vi "PhotonCamera_GetLatestResult_OLD.vi"(6 "EstimatedDataAndSampleLatency (Sec)":dbl=0.05 format="%#_13g", 8 "Pass_Through_Time":dbl=-1.0 format="%33.4f", 9 "BaseNTName":string="/photonvision", 11 "CameraName":string) -> (0 "error out":errorcluster, 1 "New Data":bool, 2 "HasTargets":bool, 3 "PipelineResult":T1={"Targets"=[], "PhotonMultiTargetPNPResult"={"PhotonPNPResult"={"IsPresent"=FALSE, "bestReprojErr"=0.0, "altReprojErr"=0.0, "ambiguity"=0.0, "Best"={"TRANSLATION3D"={"X"=0.0, "Y"=0.0, "Z"=0.0}, "ROTATION3D"={"Q_quaternion"={"R"=1.0, "V"=[0.0, 0.0, 0.0]}}, "XF"=FALSE}, "Alt"={"TRANSLATION3D"={"X"=0.0, "Y"=0.0, "Z"=0.0}, "ROTATION3D"={"Q_quaternion"={"R"=1.0, "V"=[0.0, 0.0, 0.0]}}, "XF"=FALSE}}, "FiducialIDsUsed"=[]}, "PhotonPipelineMetadata"={"CaptureTimestampMicros"=0, "PublishTimestampMicros"=0, "SequenceID"=0, "TimeSinceLastPong"=0}} {"PhotonMultiTargetPNPResult"."PhotonPNPResult"."Alt"."TRANSLATION3D"."Z" format="%14.3f"; "PhotonMultiTargetPNPResult"."PhotonPNPResult"."Alt"."TRANSLATION3D"."Y" format="%14.3f"; "PhotonMultiTargetPNPResult"."PhotonPNPResult"."Alt"."TRANSLATION3D"."X" format="%14.3f"; "PhotonMultiTargetPNPResult"."PhotonPNPResult"."Best"."TRANSLATION3D"."Z" format="%14.3f"; "PhotonMultiTargetPNPResult"."PhotonPNPResult"."Best"."TRANSLATION3D"."Y" format="%14.3f"; "PhotonMultiTargetPNPResult"."PhotonPNPResult"."Best"."TRANSLATION3D"."X" format="%14.3f"; "Targets"."AltCameraToTarget"."TRANSLATION3D"."Z" format="%14.3f"; "Targets"."AltCameraToTarget"."TRANSLATION3D"."Y" format="%14.3f"; "Targets"."AltCameraToTarget"."TRANSLATION3D"."X" format="%14.3f"; "Targets"."BestCameraToTarget"."TRANSLATION3D"."Z" format="%14.3f"; "Targets"."BestCameraToTarget"."TRANSLATION3D"."Y" format="%14.3f"; "Targets"."BestCameraToTarget"."TRANSLATION3D"."X" format="%14.3f"})   [LabVIEW 2019, in "PhotonVisionLib.lvlib"]
doc: "Returns the latest pipeline result.\n\nInputs:\n - cameraName -- The nickname of the camera (found in the PhotonVision UI).\n - BaseNTName - string - Base Nework Table name. (Optional. Default: /photonvision )\n - PassThroughTime -- (Optional. Default: Use FPGA time.) Time. Once time is available from network tables, this won't be needed. (Seconds)\n - EstimatedDataAndSampleLatency -- Estimated Network Table packet latency. This is based on the frames per second and other communications latencies. (Optional. Default: 0.050) Once time is available from network tables, this won't be needed. \n\nOutputs:\n - PipelineResult -- The latest pipeline result data cluster\n - HasTargets -- Boolean indicating if any targets were found\n - Error Out -- Contains error information if a Network table ot other error occured."
uses:
  PhotonVisionLib.lvlib
  <vilib>/Rock Robotics/Network Tables/NT Read Raw.vi
  <vilib>/Rock Robotics/WPI/ThirdParty/JAS_Junk/TrajLib/Trajectory_Library.lvlib
  TypeDef/TargetCornerType.ctl
  TypeDef/PhotonTrackedTargetType.ctl
  TypeDef/PhotonPipelineResultType.ctl
  <vilib>/Rock Robotics/WPI/ThirdParty/JAS_Junk/TrajLib/TypeDef/TRANSLATION3D.ctl
  <vilib>/Rock Robotics/WPI/ThirdParty/JAS_Junk/TrajLib/TypeDef/QUATERNION.ctl
  <vilib>/Rock Robotics/WPI/ThirdParty/JAS_Junk/TrajLib/TypeDef/ROTATION3D.ctl
  <vilib>/Rock Robotics/WPI/ThirdParty/JAS_Junk/TrajLib/TypeDef/TRANSFORM3D.ctl
  TypeDef/PhotonPNPResultType.ctl
  TypeDef/PhotonMultiTargetPNPResultType.ctl
  TypeDef/PhotonPipelineMetadataType.ctl
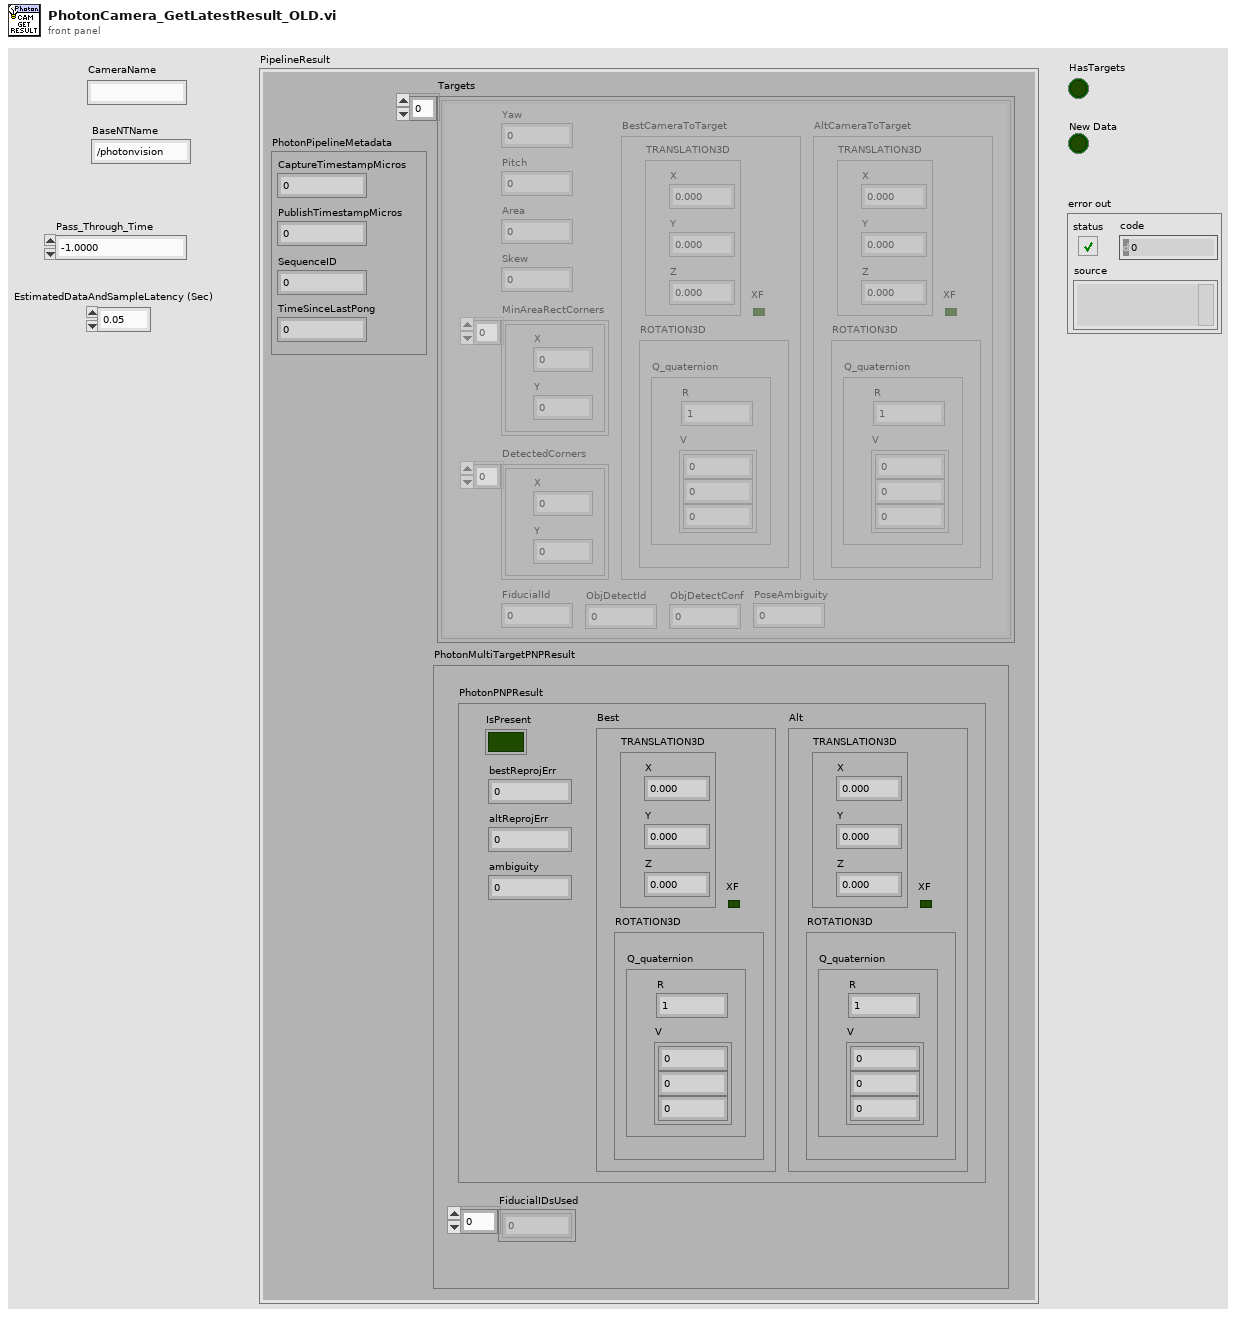
[diagram p1: front panel]
types:
  T1 = typedef "PhotonVisionLib.lvlib/PhotonPipelineResultType.ctl" = cluster{"Targets":T2[], "PhotonMultiTargetPNPResult":T8, "PhotonPipelineMetadata":T10}
  T2 = typedef "PhotonVisionLib.lvlib/PhotonTrackedTargetType.ctl" = cluster{"Yaw":dbl, "Pitch":dbl, "Area":dbl, "Skew":dbl, "MinAreaRectCorners":T3[], "BestCameraToTarget":T4, "FiducialId":i32, "AltCameraToTarget":T4, "PoseAmbiguity":dbl, "DetectedCorners":T3[], "ObjDetectId":i32, "ObjDetectConf":sgl}
  T3 = typedef "PhotonVisionLib.lvlib/TargetCornerType.ctl" = cluster{"X":dbl, "Y":dbl}
  T4 = typedef "Trajectory_Library.lvlib/TRANSFORM3D.ctl" = cluster{"TRANSLATION3D":T5, "ROTATION3D":T6, "XF":bool}
  T5 = typedef "Trajectory_Library.lvlib/TRANSLATION3D.ctl" = cluster{"X":dbl, "Y":dbl, "Z":dbl}
  T6 = typedef "Trajectory_Library.lvlib/ROTATION3D.ctl" = cluster{"Q_quaternion":T7}
  T7 = typedef "Trajectory_Library.lvlib/QUATERNION.ctl" = cluster{"R":dbl, "V":dbl[]}
  T8 = typedef "PhotonVisionLib.lvlib/PhotonMultiTargetPNPResultType.ctl" = cluster{"PhotonPNPResult":T9, "FiducialIDsUsed":i16[]}
  T9 = typedef "PhotonVisionLib.lvlib/PhotonPNPResultType.ctl" = cluster{"IsPresent":bool, "bestReprojErr":dbl, "altReprojErr":dbl, "ambiguity":dbl, "Best":T4, "Alt":T4}
  T10 = typedef "PhotonVisionLib.lvlib/PhotonPipelineMetadataType.ctl" = cluster{"CaptureTimestampMicros":i64, "PublishTimestampMicros":i64, "SequenceID":i64, "TimeSinceLastPong":i64}
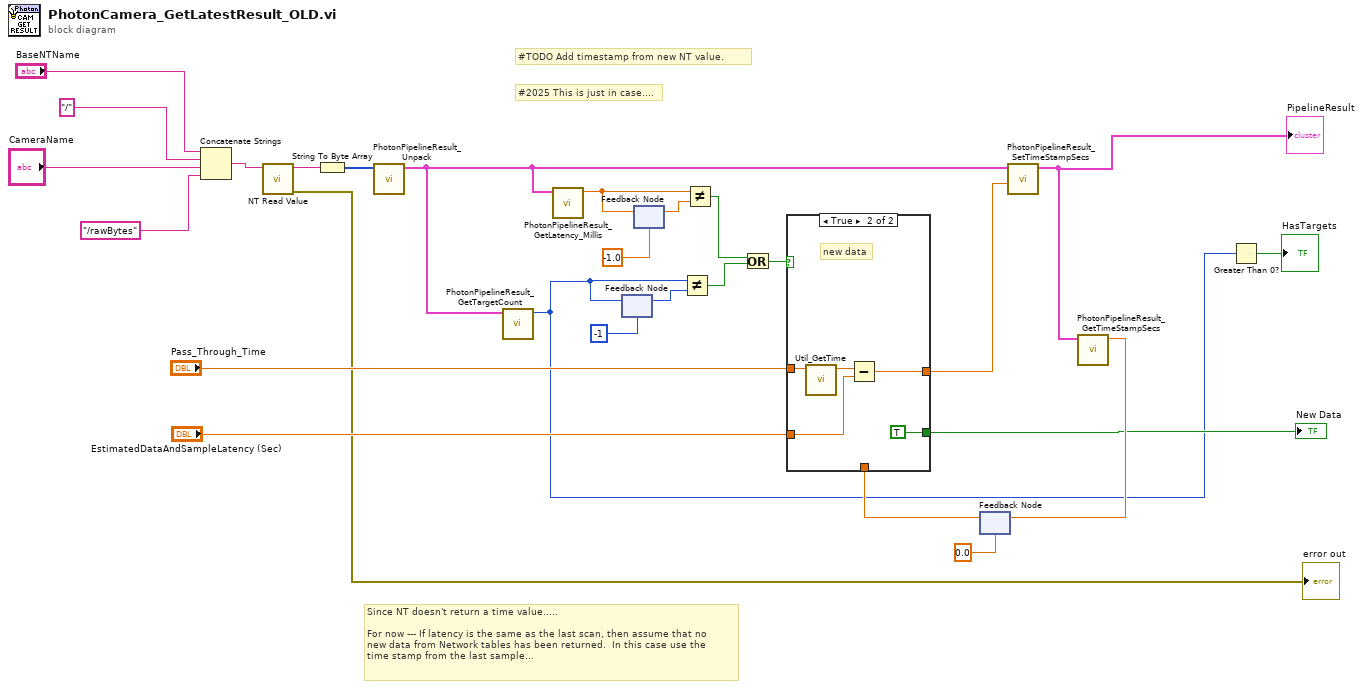
[diagram p0: block diagram]
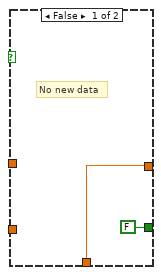
[diagram p2: hidden frame]
diagram:
  # "#2025 This is just in case...."
  # "Since NT doesn't return a time value.....\n\nFor now --- If latency is the same as the last scan, then assume that no\nnew data from Network tables has been returned.  In this case use the\ntime stamp from the last sample..."
  # "#TODO Add timestamp from new NT value."
  n1 = Concatenate Strings("BaseNTName", "/", "CameraName", "/rawBytes") -> (w25:string)
  n2 = call-poly <vilib>:"NT Read Value.vi"("name"=w25) -> ("error out"=→"error out":errorcluster, "raw"=w24:string)  [unwired: 9 in]
  n3 = String To Byte Array(string=w24) -> (unsigned byte array=w23:u8[])
  n4 = call "PhotonPipelineResult_Unpack.vi"("RawData"=w23) -> ("PhotonPipelineResult"=w2:T1)  [unwired: 10 in]
  n5 = call "PhotonPipelineResult_GetTargetCount.vi"("PhotonPipelineResult"=w2) -> ("TargetCount"=w1:i32)  [unwired: 10 in]
  n6 = call "PhotonPipelineResult_GetLatency_Millis.vi"("PhotonPipelineResult"=w2) -> ("Latency_MilliSec"=w19:dbl)  [unwired: 9 in, 1 out]
  n7 = feedback #1(-1 ("TargetCount")) -> (w9:i32)
  n8 = feedback-in #1(w1) -> ()
  n9 = feedback-in #2(w19) -> ()
  n10 = feedback #2(-1.0 ("Latency_MilliSec")) -> (w20:dbl)
  n11 = Not Equal?(x=w1, y=w9) -> (x != y?=w7:bool)
  n12 = Not Equal?(x=w19, y=w20) -> (x != y?=w10:bool)
  n13 = Or(x=w10, y=w7) -> (x .or. y?=w11:bool)
  n14 = feedback #3(0.0 ("TimeStampSec")) -> (w13:dbl)
  n15 = case shown="True" w11 {
    tunnel: "Pass_Through_Time" -> [_ w33]
    tunnel: "EstimatedDataAndSampleLatency (Sec)" -> [_ w32]
    tunnel: [w29 w30] -> w16
    tunnel: w13 -> [w29 _]
    tunnel: [FALSE TRUE] -> w6
    frame False {
      # "No new data"
    }
    frame True {
      # "new data"
      n16 = call <vilib>:"Util_GetTime.vi"("Pass_Through_Time"=w33) -> ("FPGA_Time_Seconds"=w34:dbl)  [unwired: 8 in, 2 out]
      n17 = Subtract(x=w34, y=w32) -> (x-y=w30:dbl)
    }
  }
  "New Data" <- w6
  n18 = call "PhotonPipelineResult_SetTimeStampSecs.vi"("TimeStampSec"=w16, "PhotonPipelineResult"=w2) -> ("Out PhotonPipelineResult"=w15:T1)  [unwired: 9 in]
  "PipelineResult" <- w15
  n19 = call "PhotonPipelineResult_GetTimeStampSecs.vi"("PhotonPipelineResult"=w15) -> ("TimeStampSec"=w14:dbl)  [unwired: 10 in]
  n20 = feedback-in #3(w14) -> ()
  n21 = Greater Than 0?(x=w1) -> (x > 0?=→"HasTargets":bool)
